vi "Waveform Array To Dynamic.vi"(4 "Input":waveform(dbl)[](array[waveform])) -> (1 "Output":dynamicdata(waveform))   [LabVIEW 2020]
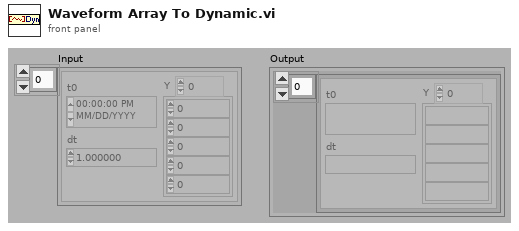
[diagram p1: front panel]
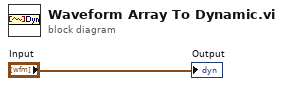
[diagram p0: block diagram]
diagram:
  "Output" <- "Input"
